vi "Main Module.vi"(8 "Error In":errorcluster) -> (0 "Error Out":errorcluster)   [LabVIEW 2015, in "Config DB.lvlib"]
uses:
  Config DB.lvlib
  Private Controls/DB Data.ctl
  Private Controls/Module Data Cluster.ctl
  Private Controls/Module Action.ctl
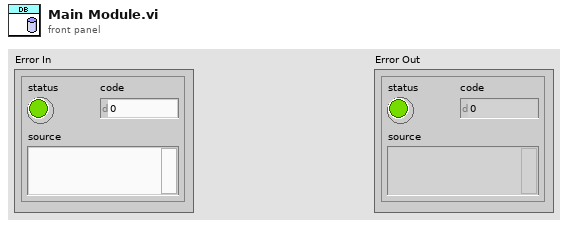
[diagram p1: front panel]
types:
  T1 = typedef "Config DB.lvlib/DB Data.ctl" = cluster{"Wash Step":string, "Station":string, "Step Duration":u32}
  T2 = typedef "Config DB.lvlib/Module Data Cluster.ctl" = cluster{"Data":variant, "Action":T3}
  T3 = typedef "Config DB.lvlib/Module Action.ctl" = enum16{"Init", "Close", "Error"}
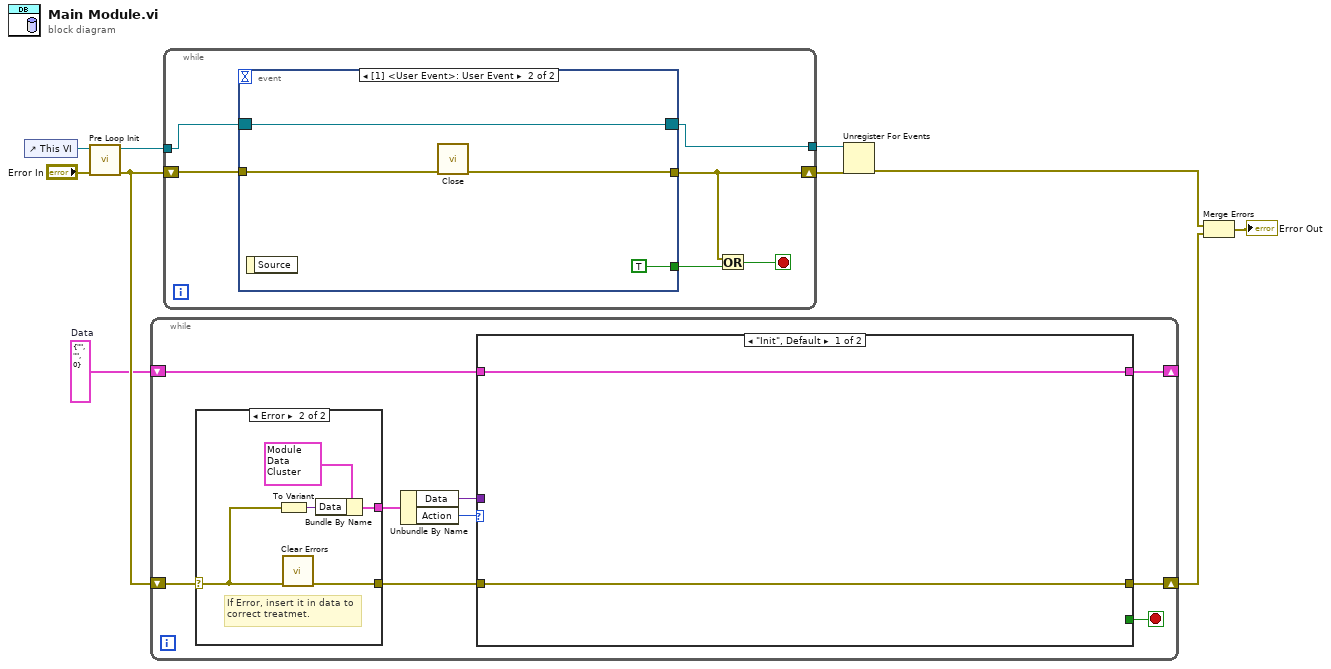
[diagram p0: block diagram]
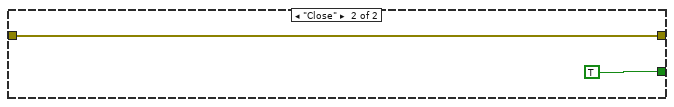
[diagram p2: hidden frame]
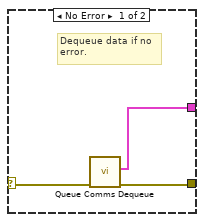
[diagram p3: hidden frame]
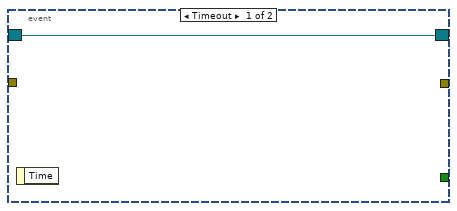
[diagram p4: hidden frame]
diagram:
  w1 = T1 {"Wash Step"="", "Station"="", "Step Duration"=0}  # Data
  n1 = control-ref of="This VI"() -> (w9:refnum<vi>)
  n2 = call "Pre Loop Init.vi"("Error In"="Error In", "This VI"=w9) -> ("Error Out"=w5:errorcluster, "Event Registration Refnum"=w8:refnum<event-registration>)  [unwired: 8 in]
  n3 = while {
    shift-right: [w13] -> w3
    shift-left: w5 -> [w19]
    shift-right: [w11] -> _
    shift-left: w1 -> [w12]
    stop <- w14 stop-if-true
    n4 = case shown="Error" w19 {
      selector: w19 -> [w26 w29]
      tunnel: [w25 w28] -> w16
      tunnel: [w24 w27] -> w18
      frame No Error {
        # "Dequeue data if no\nerror."
        n5 = call "Queue Comms Dequeue.vi"("Error In"=w26) -> ("Error Out"=w25:errorcluster, "Message Data"=w24:T2)  [unwired: 9 in]
      }
      frame Error {
        # "If Error, insert it in data to\ncorrect treatmet."
        n6 = To Variant(anything=w29) -> (Variant=w30:variant)
        n7 = call <vilib>:"Clear Errors.vi"("error in (no error)"=w29) -> ("error out"=w28:errorcluster)  [unwired: 5 in, 1 out]
        n8 = Bundle By Name(cluster=T2 {"Data"=variant, "Action"=enum."Error"} ("Message Data"), "Data"=w30) -> (w27:T2)
      }
    }
    n9 = Unbundle By Name(w18) -> ("Data"=w15:variant, "Action"=w17:T3)
    n10 = case shown="\"Init\", Default" w17 {
      tunnel: w16 -> [w21 w22]
      tunnel: w15 -> [_ _]
      tunnel: [_ TRUE] -> w14
      tunnel: [w21 w22] -> w13
      tunnel: w12 -> [w20 _]
      tunnel: [w20 _] -> w11
      frame "Init", Default {
      }
      frame "Close" {
      }
    }
  }
  n11 = while {
    tunnel: w8 -> [w37]
    shift-right: [w34] -> w7
    shift-left: w5 -> [w35]
    tunnel: [w32] -> w6
    stop <- w36 stop-if-true
    n12 = event shown="[1] <User Event>: User Event" {
      selector: w37 -> [w38 w42]
      dyn-events: [w38 w42] -> w32
      timeout: _ -> [_ _]
      tunnel: [_ w40] -> w34
      tunnel: w35 -> [_ w41]
      tunnel: [_ TRUE] -> w33
      event Timeout {
        n13 = event-data() -> ()  [unwired: 1 in, 1 out]
      }
      event User Event {
        n14 = event-data() -> ()  [unwired: 1 in, 1 out]
        n15 = call "Close.vi"("Error In"=w41) -> ("Error Out"=w40:errorcluster)  [unwired: 10 in]
      }
    }
    n16 = Or(x=w34, y=w33) -> (x .or. y?=w36:bool)
  }
  n17 = Unregister For Events(event registration refnum=w6, error in=w7) -> (error out=w2:errorcluster)
  n18 = Merge Errors(w2, w3) -> (→"Error Out":errorcluster)
